vi "UART Write.vi"(8 "error in (no error)":errorcluster, 11 "String":string) -> (0 "error out":errorcluster, 3 "Success?":bool)   [LabVIEW 2011]
uses:
  Libraries/uart_library.dll
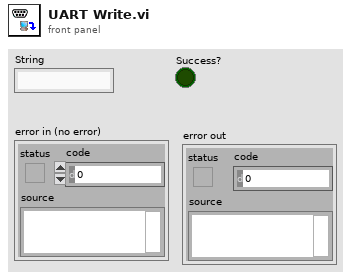
[diagram p1: front panel]
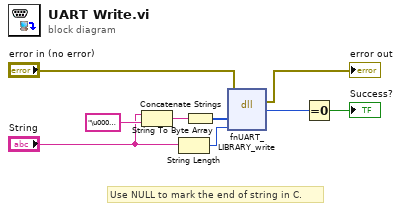
[diagram p0: block diagram]
diagram:
  # "Use NULL to mark the end of string in C."
  n1 = Concatenate Strings("String", "\u0000\u0000") -> (w3:string)
  n2 = String Length(string="String") -> (length=w9:i32)
  n3 = String To Byte Array(string=w3) -> (unsigned byte array=w1:u8[])
  n4 = dll-call lib="E:/users/tba/work_project/FW102/trunk/LabVIEW/Libraries/uart_library.dll" fn="fnUART_LIBRARY_write"(error in="error in (no error)", "Char"=w1, "Size"=w9) -> (error out=→"error out":errorcluster, "return type"=w8:i32)  [unwired: 4 in, 1 out]
  n5 = Equal To 0?(x=w8) -> (x = 0?=→"Success?":bool)
